vi "avg.vi"(0 "length":dbl[](array[numeric]), 5 "span":i32, 7 "power":dbl[](array[numeric])) -> (4 "length 2":dbl[](array[numeric]), 6 "Boolean":bool=TRUE, 8 "avg power":dbl[](array[numeric]))   [LabVIEW 2020]
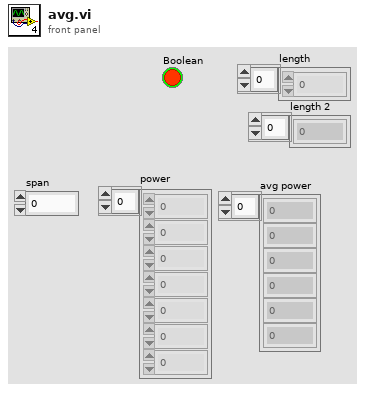
[diagram p1: front panel]
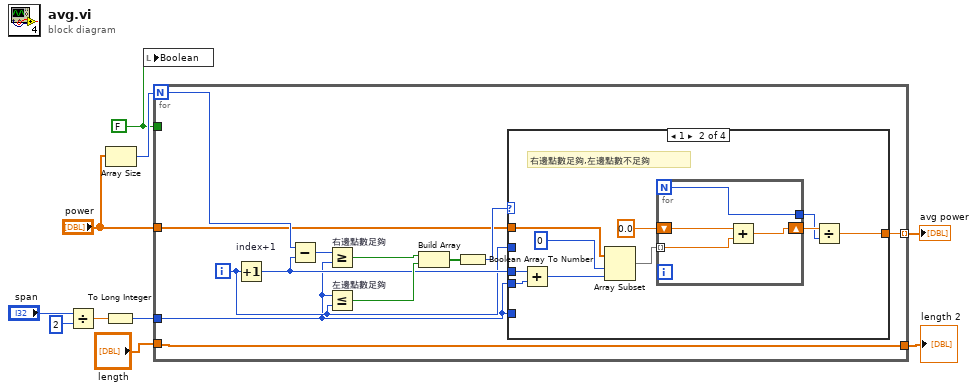
[diagram p0: block diagram]
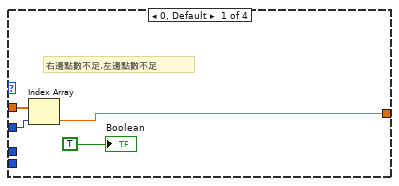
[diagram p2: hidden frame]
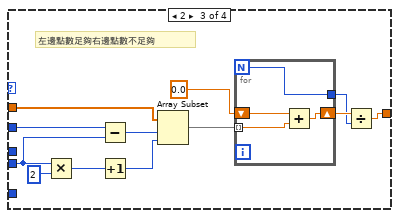
[diagram p3: hidden frame]
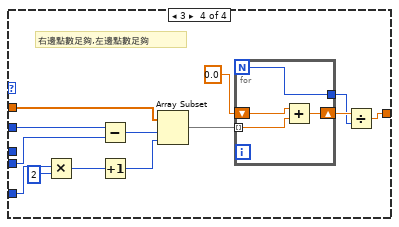
[diagram p4: hidden frame]
diagram:
  w7 = FALSE ("Boolean")
  n1 = Divide(x="span", y=2) -> (x/y=w4:dbl)
  n2 = To Long Integer(number=w4) -> (32bit integer=w3:i32)
  n3 = Array Size(array="power") -> (size(s)=w9:i32)
  n4 = local write "Boolean"(w7) -> ()
  n5 = for {
    N: w9 -> [w22]
    tunnel: "power" -> [w18]
    tunnel: w3 -> [w12]
    tunnel: [w13] -> w8 mode=indexing
    tunnel: w7 -> [_]
    tunnel: "length" -> [w11]
    tunnel: [w11] -> w1
    i -> [w14]
    n6 = Increment "index+1"(x=w14) -> (x+1=w15:i32)
    n7 = Subtract(x=w22, y=w15) -> (x-y=w21:i32)
    n8 = Greater Or Equal? "右邊點數足夠"(x=w21, y=w12) -> (x >= y?=w17:bool)
    n9 = Less Or Equal? "左邊點數足夠"(x=w12, y=w14) -> (x <= y?=w16:bool)
    n10 = Build Array(w17, w16) -> (w19:bool[])
    n11 = Boolean Array To Number(Boolean array=w19) -> (number=w20:u32)
    n12 = case shown="1" w20 {
      tunnel: w18 -> [w26 w32 w52 w69]
      tunnel: w15 -> [_ w34 _ _]
      tunnel: w12 -> [_ w33 w50 w67]
      tunnel: w14 -> [w25 _ w41 w66]
      tunnel: [w24 w27 w42 w58] -> w13
      tunnel: w12 -> [_ _ _ w57]
      frame 0, Default {
        # "右邊點數不足,左邊點數不足"
        n13 = Index Array "Index Array"(array=w26, index=w25) -> (element=w24:dbl)
        "Boolean" <- TRUE ("Boolean")
      }
      frame 1 {
        # "右邊點數足夠,左邊點數不足夠"
        n14 = Add(x=w34, y=w33) -> (x+y=w35:i32)
        n15 = Array Subset(array=w32, index=0, length=w35) -> (w31:dbl[])
        n16 = for {
          N -> [w37]
          tunnel: w31 -> [w38] mode=indexing
          shift-right: [w40] -> w29
          shift-left: 0.0 -> [w39]
          tunnel: [w37] -> w28
          n17 = Add(x=w39, y=w38) -> (x+y=w40:dbl)
        }
        n18 = Divide(x=w29, y=w28) -> (x/y=w27:dbl)
      }
      frame 2 {
        # "左邊點數足夠右邊點數不足夠"
        n19 = Multiply(x=w50, y=2) -> (x*y=w48:i32)
        n20 = Subtract(x=w41, y=w50) -> (x-y=w51:i32)
        n21 = Increment(x=w48) -> (x+1=w47:i32)
        n22 = Array Subset(array=w52, index=w51, length=w47) -> (w46:dbl[])
        n23 = for {
          N -> [w53]
          tunnel: w46 -> [w54] mode=indexing
          shift-right: [w56] -> w44
          shift-left: 0.0 -> [w55]
          tunnel: [w53] -> w43
          n24 = Add(x=w55, y=w54) -> (x+y=w56:dbl)
        }
        n25 = Divide(x=w44, y=w43) -> (x/y=w42:dbl)
      }
      frame 3 {
        # "右邊點數足夠,左邊點數足夠"
        n26 = Multiply(x=w57, y=2) -> (x*y=w64:i32)
        n27 = Subtract(x=w66, y=w67) -> (x-y=w68:i32)
        n28 = Increment(x=w64) -> (x+1=w63:i32)
        n29 = Array Subset "Array Subset"(array=w69, index=w68, length=w63) -> (w60:dbl[])
        n30 = for {
          N -> [w70]
          tunnel: w60 -> [w71] mode=indexing
          shift-right: [w73] -> w62
          shift-left: 0.0 -> [w72]
          tunnel: [w70] -> w61
          n31 = Add(x=w72, y=w71) -> (x+y=w73:dbl)
        }
        n32 = Divide(x=w62, y=w61) -> (x/y=w58:dbl)
      }
    }
  }
  "avg power" <- w8
  "length 2" <- w1
